vi "Config-Sweep-Primary Sour.vi"(0 "VISA session":refnum<visa-resource-name>, 1 "stop":dbl=1.0 format="%^.4e", 3 "start":dbl format="%^.4e", 5 "sweep spacing (linear: 0)":u16(ring) items=["linear", "log 10", "log 25", "log 50"], 7 "step (linear only)":dbl=0.01 format="%^.4e", 9 "sweep mode":bool, 11 "error in (no error)":errorcluster, 12 "compliance":dbl=0.1 format="%^.2e", 14 "power compliance (0 = OFF)":dbl format="%^.2e") -> (4 "VISA resource name out":refnum<visa-resource-name>, 15 "error out":errorcluster)   [LabVIEW 2016, in "Agilent 415X Series.lvlib"]
doc: "This VI configures the primary sweep source (VAR1) for a sweep mode measurement. \n* This VI does not perform error checking on MEASUREMENT MODE or UNIT TYPE of VAR1, therefore it is the application programmer's responsibility to make certain this VI is used in the proper mode."
uses:
  Agilent 415X Series.lvlib
panel:
  # "(W)"
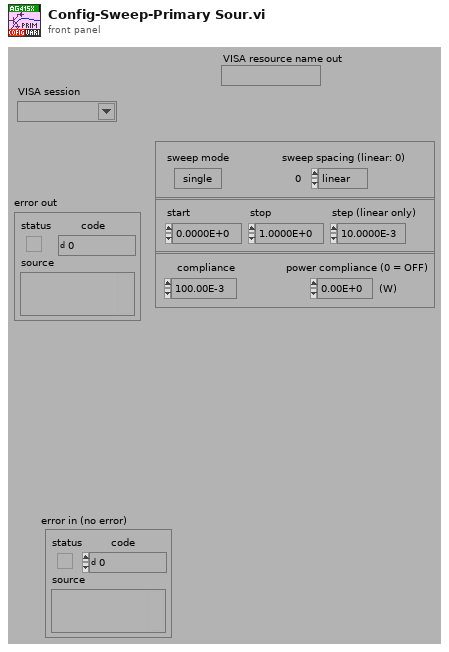
[diagram p1: front panel]
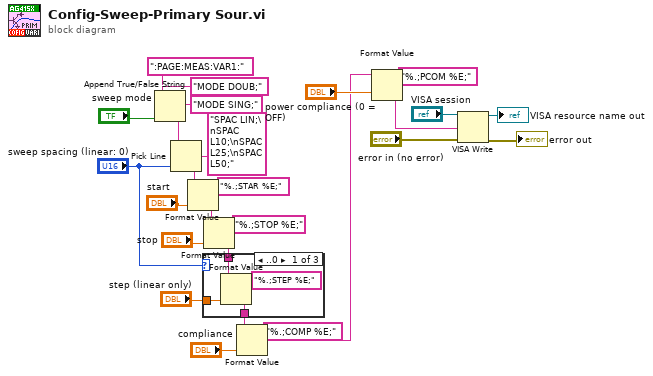
[diagram p0: block diagram]
diagram:
  n1 = Append True/False String(1:"sweep mode", 2:"MODE SING;", 3:"MODE DOUB;", 4:":PAGE:MEAS:VAR1:") -> (0:w5:string)
  n2 = Pick Line(string ("")=w5, multi-line string="SPAC LIN;\nSPAC L10;\nSPAC L25;\nSPAC L50;", line index="sweep spacing (linear: 0)") -> (output string=w3:string)
  n3 = Format Value(string ("")=w3, format string="%.;STAR %E;", value (0)="start") -> (output string=w23:string)
  n4 = Format Value(string ("")=w23, format string="%.;STOP %E;", value (0)="stop") -> (output string=w21:string)
  n5 = case shown="..0" "sweep spacing (linear: 0)" {
    tunnel: w21 -> [w29 w31 w32]
    tunnel: [w28 w31 w32] -> w18
    tunnel: "step (linear only)" -> [w27 _ _]
    frame ..0 {
      # "linear"
      n6 = Format Value(string ("")=w29, format string="%.;STEP %E;", value (0)=w27) -> (output string=w28:string)
    }
    frame 1 {
      # "log"
    }
    frame 2.. {
      # "log"
    }
  }
  n7 = Format Value(string ("")=w18, format string="%.;COMP %E;", value (0)="compliance") -> (output string=w15:string)
  n8 = Format Value(string ("")=w15, format string="%.;PCOM %E;", value (0)="power compliance (0 = OFF)") -> (output string=w14:string)
  n9 = VISA Write(VISA resource name="VISA session", write buffer=w14, error in (no error)="error in (no error)") -> (VISA resource name out=→"VISA resource name out":refnum<visa-resource-name>, error out=→"error out":errorcluster)  [unwired: 1 out]
